vi "Cell I Readback.vi"(7 "Box ID":u8=1, 8 "error in (no error)":errorcluster, 10 "Channel":u16=1 min=1 max=12 step=1, 11 "CAN in":refnum<class "XNET_BS120x.lvclass">) -> (0 "error out":errorcluster, 2 "Current (mA)":dbl, 3 "CAN out":refnum<class "XNET_BS120x.lvclass">)   [LabVIEW 2021, in "BS120x Driver.lvlib" / "XNET_BS120x.lvclass"]
uses:
  XNET_BS120x.lvclass
  BS120x.lvclass
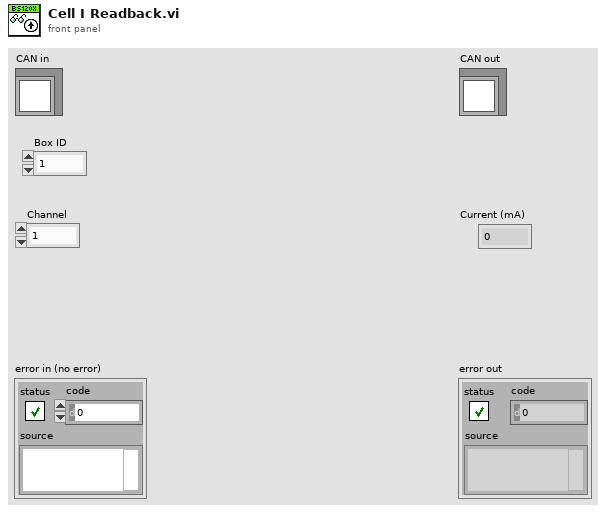
[diagram p1: front panel]
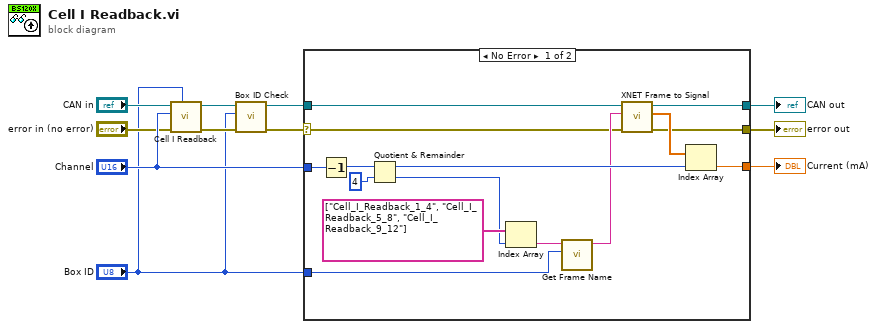
[diagram p0: block diagram]
diagram:
  n1 = call-parent "Cell I Readback.vi"("Box ID"="Box ID", "error in (no error)"="error in (no error)", "Channel"="Channel", "BS120x in"="CAN in") -> ("error out"=w3:errorcluster, "BS120x out"=w5:refnum<class "XNET_BS120x.lvclass">)  [unwired: 5 in, 1 out]
  n2 = call "Box ID Check.vi"("error in (no error)"=w3, "Box ID"="Box ID", "CAN in"=w5) -> ("error out"=w6:errorcluster, "CAN out"=w7:refnum<class "XNET_BS120x.lvclass">)  [unwired: 7 in]
  n3 = case shown="No Error" w6 {
    selector: w6 -> [w15 w27]
    tunnel: w7 -> [w22 w28]
    tunnel: [w21 w28] -> w10
    tunnel: "Channel" -> [w20 _]
    tunnel: [w19 _] -> w9
    tunnel: [w18 w27] -> w8
    tunnel: "Box ID" -> [w16 _]
    frame No Error {
      n4 = Decrement(x=w20) -> (x-1=w24:u16)
      n5 = Quotient & Remainder(x=w24, y=u16 4) -> (x-y*floor(x/y)=w25:u16, floor(x/y)=w13:u16)
      n6 = Index Array(array=string[] ["Cell_I_Readback_1_4", "Cell_I_Readback_5_8", "Cell_I_Readback_9_12"], index=w13) -> (element=w12:string)
      n7 = call "Get Frame Name.vi"("Box ID"=w16, "Frame Name"=w12) -> ("Frame Name out"=w17:string)  [unwired: 9 in]
      n8 = call "XNET Frame to Signal.vi"("error in (no error)"=w15, "Frame"=w17, "CAN in"=w22) -> ("error out"=w18:errorcluster, "signal data"=w26:dbl[], "CAN out"=w21:refnum<class "XNET_BS120x.lvclass">)  [unwired: 6 in]
      n9 = Index Array(array=w26, index=w25) -> (element=w19:dbl)
    }
    frame Error {
    }
  }
  "error out" <- w8
  "CAN out" <- w10
  "Current (mA)" <- w9
